vi "calSubtractBkg.vi"(8 "bkg end":i32, 9 "bkg start":i32, 10 "660":dbl[](array[numeric]), 11 "532":dbl[](array[numeric])) -> (2 "660 Substracted":dbl[](array[numeric]), 3 "532 Subtracted":dbl[](array[numeric]))   [LabVIEW 2011]
uses:
  <vilib>/Analysis/NI_AALBase.lvlib
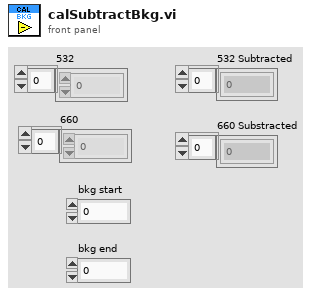
[diagram p1: front panel]
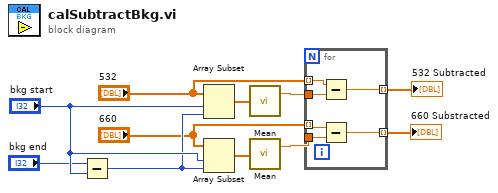
[diagram p0: block diagram]
diagram:
  n1 = Subtract(x="bkg end", y="bkg start") -> (x-y=w6:i32)
  n2 = Array Subset(array="532", index="bkg start", length=w6) -> (w8:dbl[])
  n3 = Array Subset(array="660", index="bkg start", length=w6) -> (w9:dbl[])
  n4 = call <vilib>:"Mean.vi"("X"=w8) -> ("mean"=w10:dbl)  [unwired: 1 out]
  n5 = call <vilib>:"Mean.vi"("X"=w9) -> ("mean"=w11:dbl)  [unwired: 1 out]
  n6 = for {
    tunnel: w11 -> [w17]
    tunnel: w10 -> [w16]
    tunnel: "532" -> [w15] mode=indexing
    tunnel: "660" -> [w14] mode=indexing
    tunnel: [w13] -> w2 mode=indexing
    tunnel: [w12] -> w1 mode=indexing
    n7 = Subtract(x=w15, y=w16) -> (x-y=w13:dbl)
    n8 = Subtract(x=w14, y=w17) -> (x-y=w12:dbl)
  }
  "532 Subtracted" <- w2
  "660 Substracted" <- w1
